vi "Unlock ECU.vi"(8 "error in (no error)":errorcluster, 11 "Node Ptr":T2 format="%.0x") -> (0 "error out":errorcluster)   [LabVIEW 2019, in "Diagnostics Addon System Explorer.lvlib"]
uses:
  Diagnostics Addon System Explorer.lvlib
  <vilib>/NI VeriStand/Custom Device API/Custom Device API.lvlib
  Types/FG.Action.ctl
  <vilib>/NI VeriStand/Custom Device API/Custom Device Item Ref.ctl
  Shared/Types/Security.Type.ctl
  Shared/Diagnostics Addon Shared.lvlib
panel:
  in  "Access Mode":u8 format="%.0x"
  in  "Seed Key DLL Path":path
  in  "Type":T1
  in  "Master Key":string
  in  "Header":cluster{"Section Name":string}={"Section Name"="Security Settings"}
  in  "SHDocVw.IWebBrowser":refnum<k7>(container)
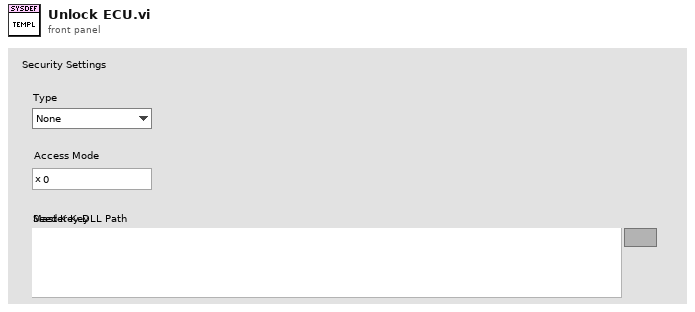
[diagram p1: front panel]
types:
  T1 = typedef "Diagnostics Addon Shared.lvlib/Security.Type.ctl" = enum16{"None", "DLL", "MasterKey"}
  T2 = typedef "Custom Device API.lvlib/Custom Device Item Ref.ctl" = u64
  T3 = typedef "Diagnostics Addon System Explorer.lvlib/FG.Action.ctl" = enum16{"Get", "Set"}
  T4 = typedef "Custom Device API.lvlib/Custom Device Item Info.ctl" = cluster{"Name":string, "Is Channel":bool, "GUID":string, "Is Waveform":bool}
  T5 = typedef "Diagnostics Addon Shared.lvlib/Security.ctl" = cluster{"Type":T1, "Source DLL Path":path, "Target DLL Path":path, "Security Level":u8, "Master Key":string}
  T6 = typedef "Custom Device API.lvlib/Custom Device Commands.ctl" = enum16{"Default", "Item renamed", "Shutdown", "Dynamic button pressed"}
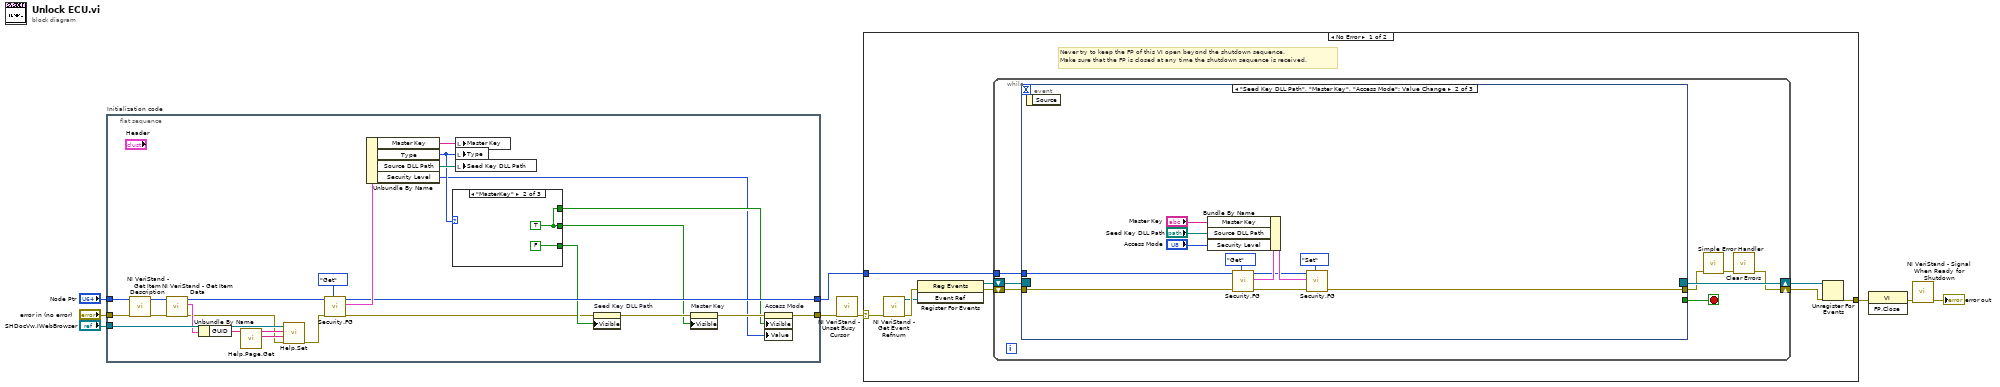
[diagram p0: block diagram]
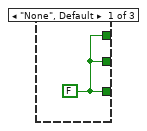
[diagram p2: hidden frame]
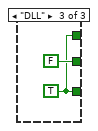
[diagram p3: hidden frame]
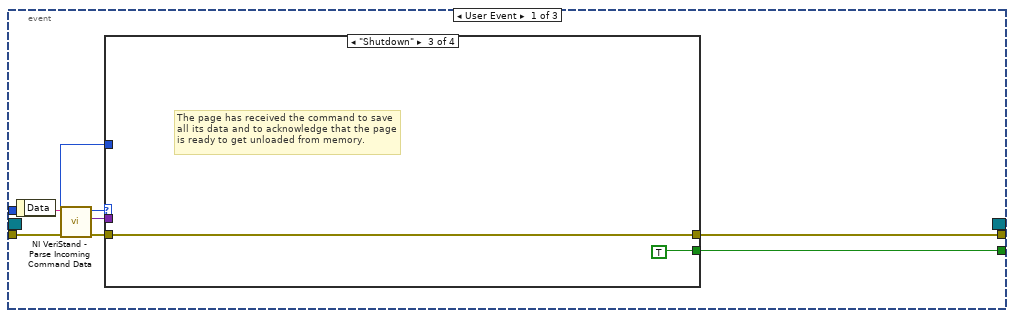
[diagram p4: hidden frame]
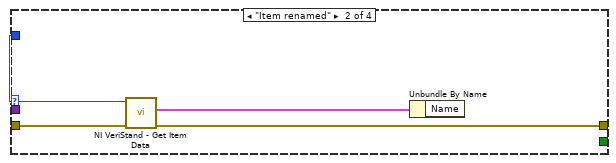
[diagram p6: hidden frame]
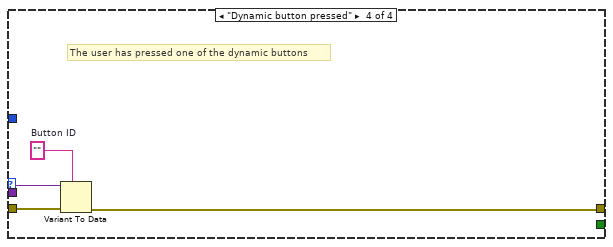
[diagram p7: hidden frame]
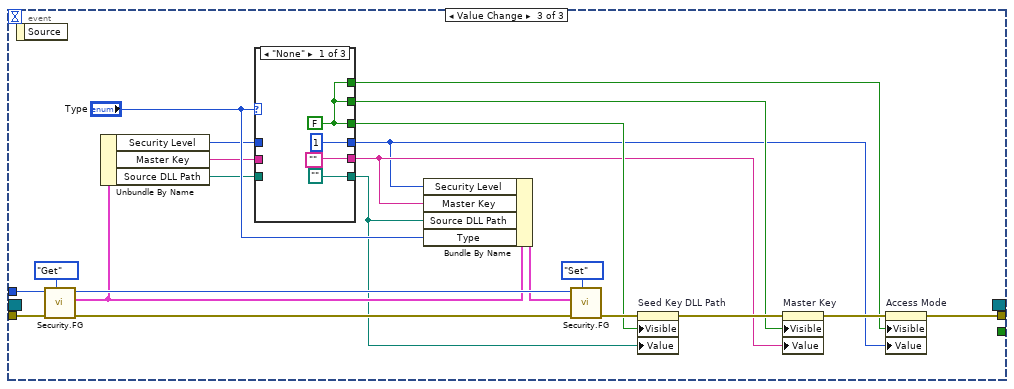
[diagram p8: hidden frame]
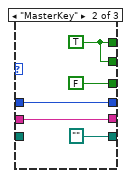
[diagram p9: hidden frame]
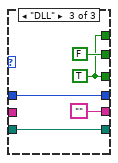
[diagram p10: hidden frame]
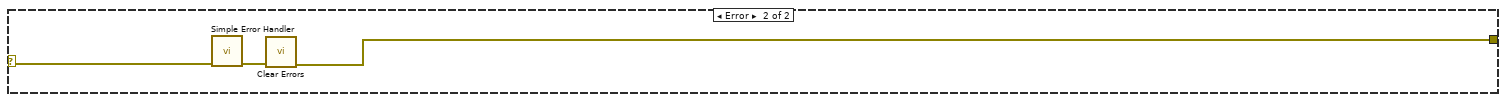
[diagram p11: hidden frame]
diagram:
  n1 = flat-sequence "Initialization code" {
    tunnel: "error in (no error)" -> [w14]
    tunnel: "Node Ptr" -> [w18]
    tunnel: [w22] -> w5
    tunnel: [w29] -> w2
    tunnel: "SHDocVw.IWebBrowser" -> [w33]
    frame #0 {
      n2 = call <vilib>:"NI VeriStand - Get Item Description.vi"("error in (no error)"=w14, "Item Ref in"=w18) -> ("error out"=w34:errorcluster, "Item Ref out"=w35:T2)  [unwired: 8 out]
      n3 = call <vilib>:"NI VeriStand - Get Item Data.vi"("error in (no error)"=w34, "Item Ref in"=w35) -> ("error out"=w11:errorcluster, "Item Info"=w13:T4, "Item Ref out"=w19:T2)  [unwired: 7 out]
      n4 = Unbundle By Name(w13) -> ("GUID"=w12:string)
      n5 = call "Help.Page.Get.vi"("GUID"=w12) -> ("HTML File"=w15:string, "Main CHM File"=w16:string)  [unwired: 9 in]
      n6 = call "Help.Set.vi"("error in (no error)"=w11, "HTML File"=w15, "Main CHM File"=w16, "SHDocVw.IWebBrowser2"=w33) -> ("error out"=w10:errorcluster)  [unwired: 7 in]
      n7 = call "Security.FG.vi"("Action"=FG.Action."Get", "error in (no error)"=w10, "Device Item Ref in"=w19) -> ("error out"=w17:errorcluster, "Security"=w32:T5, "Device Item Ref out"=w29:T2)  [unwired: 6 in]
      n8 = Unbundle By Name(w32) -> ("Master Key"=w24:string, "Type"=w27:T1, "Source DLL Path"=w30:path, "Security Level"=w20:u8)
      n9 = case shown="\"MasterKey\"" w27 {
        tunnel: [w36 FALSE w39] -> w26
        tunnel: [w36 w37 FALSE] -> w25
        tunnel: [w36 w37 w39] -> w21
        frame "None", Default {
          w36 = FALSE
        }
        frame "MasterKey" {
          w37 = TRUE
        }
        frame "DLL" {
          w39 = TRUE
        }
      }
      n10 = local write "Master Key"(w24) -> ()
      n11 = local write "Type"(w27) -> ()
      n12 = local write "Seed Key DLL Path"(w30) -> ()
      n13 = property on="Seed Key DLL Path" class="Path"(error in=w17, "Visible"=w26) -> (error out=w28:errorcluster)  [unwired: 1 in, 1 out]
      n14 = property on="Master Key" class="Str"(error in=w28, "Visible"=w25) -> (error out=w23:errorcluster)  [unwired: 1 in, 1 out]
      n15 = property on="Access Mode" class="DigNum (strict)"(error in=w23, "Visible"=w21, "Value"=w20) -> (error out=w22:errorcluster)  [unwired: 1 in, 1 out]
    }
  }
  n16 = call <vilib>:"NI VeriStand - Unset Busy Cursor.vi"("error in (no error)"=w5) -> ("error out"=w4:errorcluster)  [unwired: 10 out]
  n17 = case shown="No Error" w4 {
    selector: w4 -> [w41 w127]
    tunnel: [w46 w125] -> w9
    tunnel: w2 -> [w42 _]
    frame No Error {
      # "Never try to keep the FP of this VI open beyond the shutdown sequence.\nMake sure that the FP is closed at any time the shutdown sequence is received."
      n18 = call <vilib>:"NI VeriStand - Get Event Refnum.vi"("error in (no error)"=w41) -> ("error out"=w49:errorcluster, "Event Ref"=w45:refnum<user-event>)  [unwired: 9 out]
      n19 = register-events(error in=w49, w45) -> (reference out=w43:refnum<event-registration>, error out=w44:errorcluster)  [unwired: 1 in]
      n20 = while {
        tunnel: w42 -> [w53]
        shift-right: [w50] -> w47
        shift-left: w44 -> [w56]
        shift-right: [w57] -> w48
        shift-left: w43 -> [w55]
        stop <- w54 stop-if-true
        n21 = event shown="[1] \"Seed Key DLL Path\", \"Master Key\", \"Access Mode\": Value Change" {
          selector: w55 -> [_ _ _]
          dyn-events: [_ _ _] -> w57
          timeout: _ -> [_ _ _]
          tunnel: w56 -> [w65 w88 w110]
          tunnel: [w61 _ _] -> w54
          tunnel: [w60 w81 w92] -> w52
          tunnel: w53 -> [w59 w87 w109]
          event User Event {
            n22 = event-data() -> ("Data"=w64:string)  [unwired: 1 out]
            n23 = call <vilib>:"NI VeriStand - Parse Incoming Command Data.vi"("error in (no error)"=w65, "Incoming data"=w64) -> ("error out"=w63:errorcluster, "Outgoing data"=w58:variant, "Action"=w62:T6)  [unwired: 7 out]
            n24 = case shown="\"Shutdown\"" w62 {
              tunnel: w63 -> [w66 w70 w71 w76]
              tunnel: [_ _ TRUE _] -> w61
              tunnel: [w66 w67 w71 w73] -> w60
              tunnel: w59 -> [_ w69 _ _]
              tunnel: w58 -> [_ _ _ w75]
              frame "Default", Default {
              }
              frame "Item renamed" {
                n25 = call <vilib>:"NI VeriStand - Get Item Data.vi"("error in (no error)"=w70, "Item Ref in"=w69) -> ("error out"=w67:errorcluster, "Item Info"=w68:T4)  [unwired: 8 out]
                n26 = Unbundle By Name(w68) -> ()  [unwired: 1 out]
              }
              frame "Shutdown" {
                # "The page has received the command to save all its data and to acknowledge that the page is ready to get unloaded from memory."
              }
              frame "Dynamic button pressed" {
                w74 = ""  # Button ID
                # "The user has pressed one of the dynamic buttons"
                n27 = Variant To Data(error in=w76, type=w74, Variant=w75) -> (error out=w73:errorcluster)  [unwired: 1 out]
              }
            }
          }
          event "Seed Key DLL Path", "Master Key", "Access Mode": Value Change {
            n28 = event-data() -> ()  [unwired: 2 out]
            n29 = call "Security.FG.vi"("Action"=FG.Action."Get", "error in (no error)"=w88, "Device Item Ref in"=w87) -> ("error out"=w83:errorcluster, "Security"=w86:T5, "Device Item Ref out"=w82:T2)  [unwired: 6 in]
            n30 = Bundle By Name(cluster=w86, "Master Key"="Master Key", "Source DLL Path"="Seed Key DLL Path", "Security Level"="Access Mode") -> (w84:T5)
            n31 = call "Security.FG.vi"("Action"=FG.Action."Set", "error in (no error)"=w83, "Security"=w84, "Device Item Ref in"=w82) -> ("error out"=w81:errorcluster)  [unwired: 5 in, 2 out]
          }
          event Value Change {
            n32 = event-data() -> ()  [unwired: 2 out]
            n33 = call "Security.FG.vi"("Action"=FG.Action."Get", "error in (no error)"=w110, "Device Item Ref in"=w109) -> ("error out"=w107:errorcluster, "Security"=w98:T5, "Device Item Ref out"=w106:T2)  [unwired: 6 in]
            n34 = Unbundle By Name(w98) -> ("Security Level"=w90:u8, "Master Key"=w95:string, "Source DLL Path"=w97:path)
            n35 = case shown="\"None\"" "Type" {
              tunnel: [w112 FALSE w121] -> w100
              tunnel: [w112 w116 FALSE] -> w99
              tunnel: w97 -> [_ _ w123]
              tunnel: [path "" path "" w123] -> w96
              tunnel: ["" w117 ""] -> w94
              tunnel: w95 -> [_ w117 _]
              tunnel: [w112 w116 w121] -> w91
              tunnel: w90 -> [_ w115 w120]
              tunnel: [u8 1 w115 w120] -> w89
              frame "None" {
                w112 = FALSE
              }
              frame "MasterKey" {
                w116 = TRUE
              }
              frame "DLL" {
                w121 = TRUE
              }
            }
            n36 = Bundle By Name(cluster=w98, "Security Level"=w89, "Master Key"=w94, "Source DLL Path"=w96, "Type"="Type") -> (w104:T5)
            n37 = call "Security.FG.vi"("Action"=FG.Action."Set", "error in (no error)"=w107, "Security"=w104, "Device Item Ref in"=w106) -> ("error out"=w102:errorcluster)  [unwired: 5 in, 2 out]
            n38 = property on="Seed Key DLL Path" class="Path"(error in=w102, "Visible"=w100, "Value"=w96) -> (error out=w103:errorcluster)  [unwired: 1 in, 1 out]
            n39 = property on="Master Key" class="Str"(error in=w103, "Visible"=w99, "Value"=w94) -> (error out=w93:errorcluster)  [unwired: 1 in, 1 out]
            n40 = property on="Access Mode" class="DigNum (strict)"(error in=w93, "Visible"=w91, "Value"=w89) -> (error out=w92:errorcluster)  [unwired: 1 in, 1 out]
          }
        }
        n41 = call <vilib>:"Simple Error Handler.vi"("error in (no error)"=w52) -> ("error out"=w51:errorcluster)  [unwired: 1 in, 7 out]
        n42 = call <vilib>:"Clear Errors.vi"("error in (no error)"=w51) -> ("error out"=w50:errorcluster)  [unwired: 1 in, 5 out]
      }
      n43 = Unregister For Events(event registration refnum=w48, error in=w47) -> (error out=w46:errorcluster)
    }
    frame Error {
      n44 = call <vilib>:"Simple Error Handler.vi"("error in (no error)"=w127) -> ("error out"=w126:errorcluster)  [unwired: 1 in, 7 out]
      n45 = call <vilib>:"Clear Errors.vi"("error in (no error)"=w126) -> ("error out"=w125:errorcluster)  [unwired: 1 in, 5 out]
    }
  }
  n46 = invoke class="VI" method="FP.Close"(error in=w9) -> (error out=w8:errorcluster)  [unwired: 2 in, 2 out]
  n47 = call <vilib>:"NI VeriStand - Signal When Ready for Shutdown.vi"("error in (no error)"=w8) -> ("error out"=→"error out":errorcluster)  [unwired: 10 out]
